vi "UDP_fTales.vi"() -> ()   [LabVIEW 2016]
panel:
  in  "stop":bool
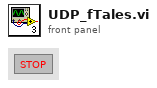
[diagram p1: front panel]
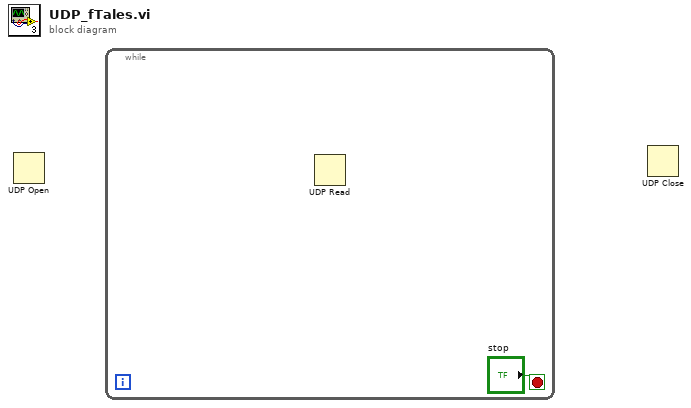
[diagram p0: block diagram]
diagram:
  n1 = UDP Open() -> ()  [unwired: 5 in, 3 out]
  n2 = while {
    stop <- "stop" stop-if-true
    n3 = UDP Read() -> ()  [unwired: 4 in, 5 out]
  }
  n4 = UDP Close() -> ()  [unwired: 2 in, 2 out]
